vi "DPO_7K_WaitForAcquisition.vi"(8 "Error In":errorcluster, 10 "Number of Waveforms":i32, 11 "VISA resource name in":refnum<visa-resource-name>) -> (0 "Error Out":errorcluster, 3 "VISA resource name out":refnum<visa-resource-name>)   [LabVIEW 2020]
uses:
  <vilib>/ErrorRing/Error Ring.xnode
  <vilib>/Utility/error.llb/Error Cluster From Error Code.vi
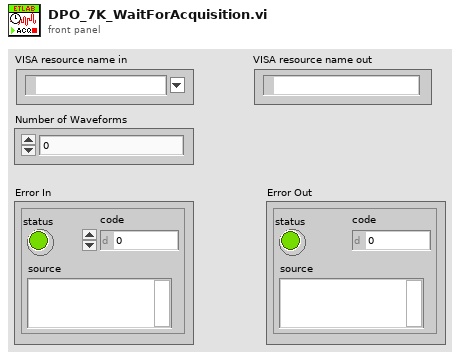
[diagram p1: front panel]
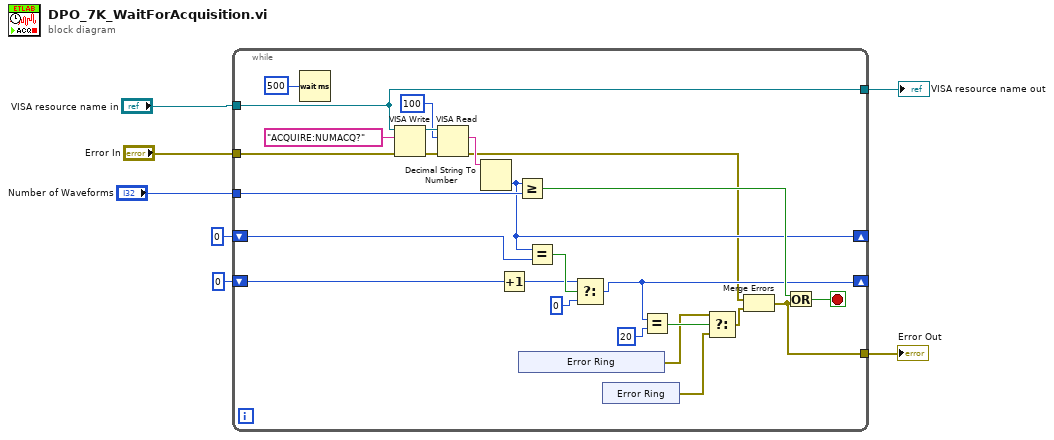
[diagram p0: block diagram]
diagram:
  n1 = while {
    tunnel: "VISA resource name in" -> [w23]
    tunnel: [w8] -> w7
    tunnel: "Number of Waveforms" -> [w26]
    tunnel: [w23] -> w3
    tunnel: "Error In" -> [w22]
    shift-right: [w21] -> _
    shift-left: 0 -> [w20]
    shift-right: [w15] -> _
    shift-left: 0 -> [w16]
    stop <- w24 stop-if-true
    n2 = Wait (ms)(milliseconds to wait=u32 500) -> ()  [unwired: 1 out]
    n3 = VISA Write(VISA resource name=w23, write buffer="ACQUIRE:NUMACQ?", error in (no error)=w22) -> (VISA resource name out=w30:refnum<visa-resource-name>, error out=w31:errorcluster)  [unwired: 1 out]
    n4 = VISA Read(VISA resource name=w30, byte count=u32 100, error in (no error)=w31) -> (read buffer=w28:string, error out=w9:errorcluster)  [unwired: 2 out]
    n5 = Decimal String To Number(string=w28) -> (number=w21:i32)  [unwired: 2 in, 1 out]
    n6 = Increment(x=w16) -> (x+1=w17:i32)
    n7 = Greater Or Equal?(x=w21, y=w26) -> (x >= y?=w25:bool)
    n8 = xnode "Error Ring"() -> ("error out"=w12:errorcluster)
    n9 = Equal?(x=w21, y=w20) -> (x = y?=w19:bool)
    n10 = Select(t=w17, s=w19, f=0) -> (s? t:f=w15:i32)
    n11 = xnode "Error Ring"() -> ("error out"=w11:errorcluster)
    n12 = Equal?(x=w15, y=20) -> (x = y?=w13:bool)
    n13 = Select(t=w12, s=w13, f=w11) -> (s? t:f=w10:errorcluster)
    n14 = Merge Errors(w9, w10) -> (w8:errorcluster)
    n15 = Or(x=w25, y=w8) -> (x .or. y?=w24:bool)
  }
  "Error Out" <- w7
  "VISA resource name out" <- w3
